vi "Initialise.vi"(8 "error in (no error)":errorcluster) -> (0 "error out":errorcluster, 2 "Test Actor API out":refnum<class "Test Actor API.lvclass">, 3 "Test Actor out":refnum<class "Test Actor.lvclass">)   [LabVIEW 2020, in "Test Actor.lvclass"]
uses:
  Test Actor.lvclass
  C:/Users/neilp/Desktop/Actors/Actor/Actor/Actor.lvclass
  API/Test Actor API.lvclass
  C:/Users/neilp/Desktop/Actors/Actor/API/Actor API.lvclass
  Base Actor/Actor/Actor.lvclass
  Base Actor/API/Actor API.lvclass
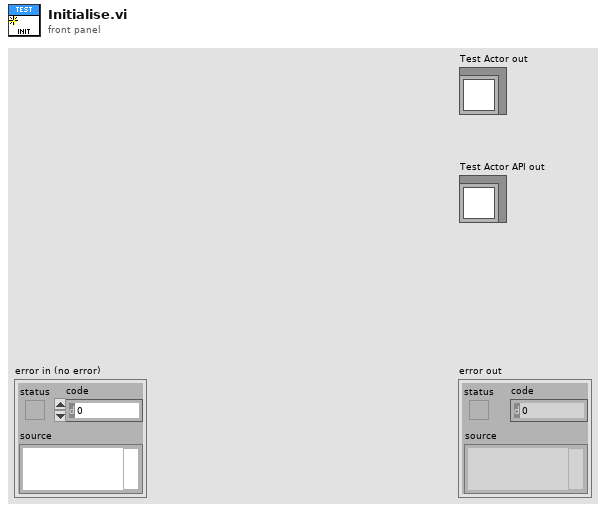
[diagram p1: front panel]
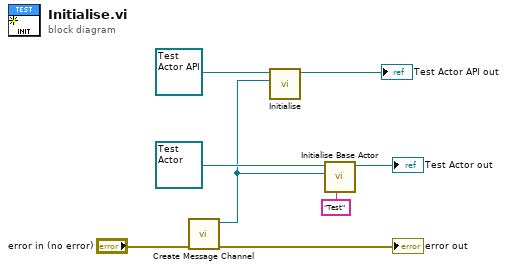
[diagram p0: block diagram]
diagram:
  n1 = call "Create Message Channel.vi"("error in (no error)"="error in (no error)") -> ("error out"=→"error out":errorcluster, "Message Channel"=w1:refnum<user-event>)  [unwired: 9 in]
  n2 = call "Initialise.vi"("Message Channel"=w1, "Actor API in"=refnum<class "Test Actor API.lvclass"> refnum ("Test Actor API.lvclass")) -> ("Actor API out"=→"Test Actor API out":refnum<class "Test Actor API.lvclass">)  [unwired: 9 in]
  n3 = call "Initialise Base Actor.vi"("Name"="Test", "Received Messages Channel"=w1, "Actor in"=refnum<class "Test Actor.lvclass"> refnum ("Test Actor.lvclass")) -> ("Actor out"=→"Test Actor out":refnum<class "Test Actor.lvclass">)  [unwired: 7 in, 1 out]
